vi "Str_Data.vi"(1 "Err str":string, 2 "Msg":T1 {"ID" format="%x"; "MSGTYPE" items=["STATUS"=128, "EXTENDED"=2, "RTR"=1, "DATA MSG"=0]; "aDATA" format="%x"}, 3 "string":string) -> (0 "str out":string)   [LabVIEW 2010]
panel:
  out "str out 2":string
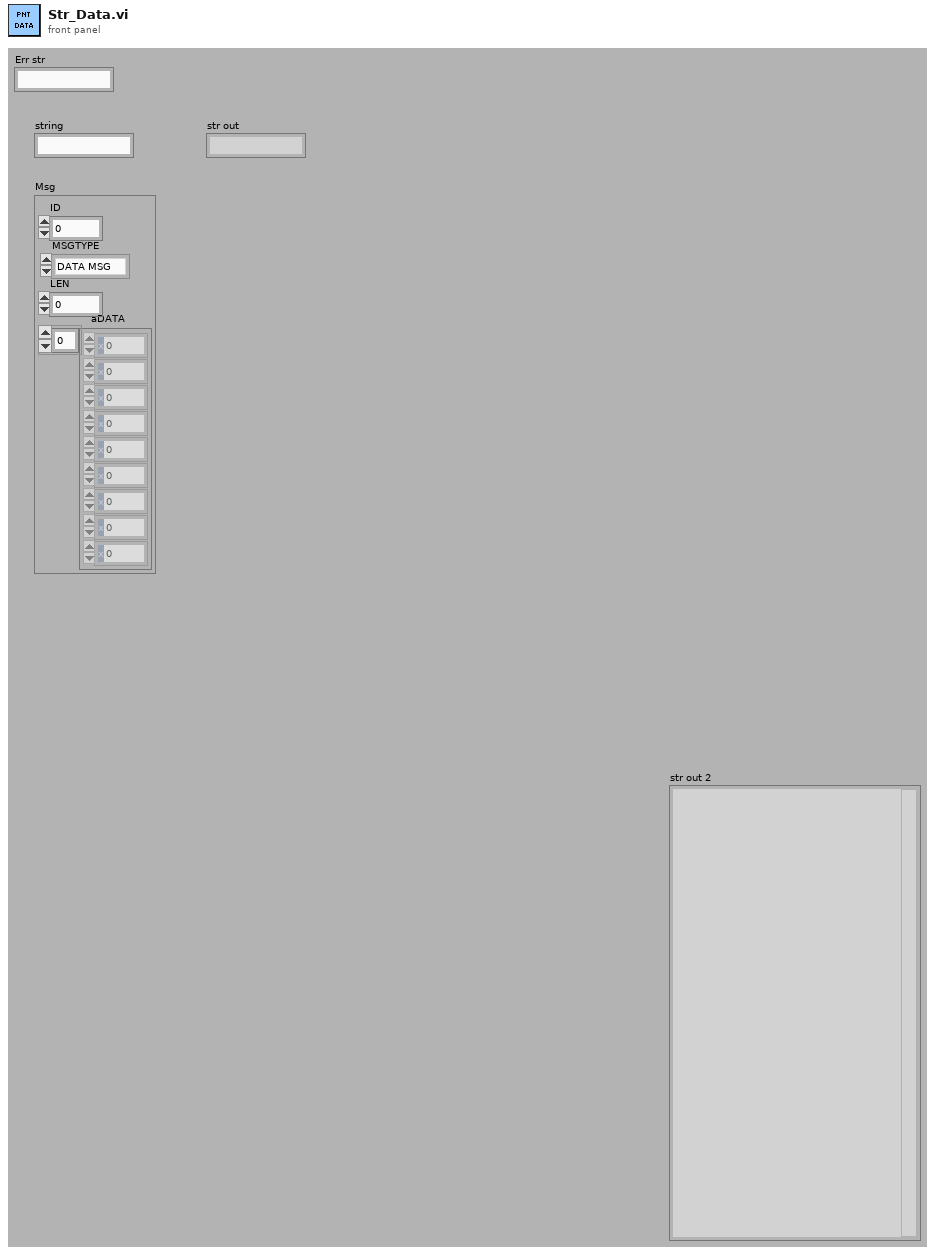
[diagram p1: front panel]
types:
  T1 = cluster{"ID":u32, "MSGTYPE":u8, "LEN":u8, "aDATA":u8[]}
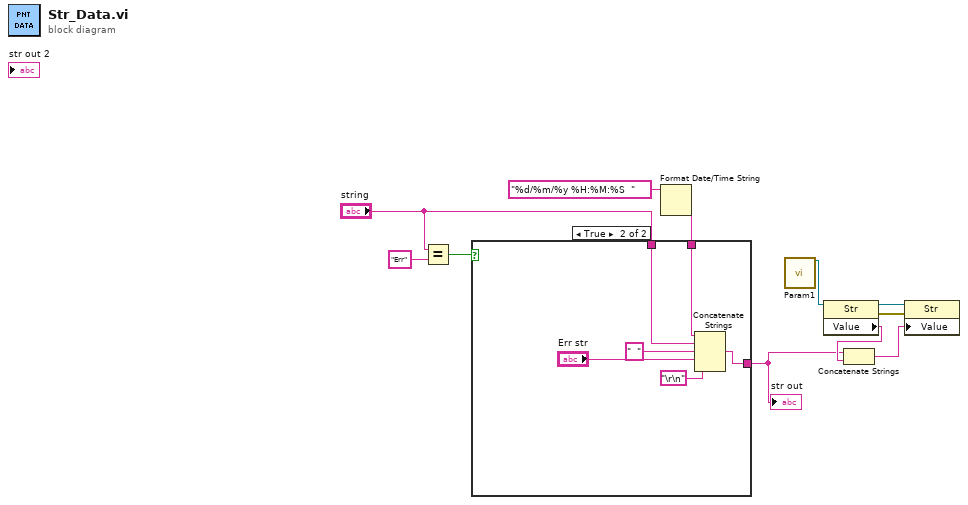
[diagram p0: block diagram]
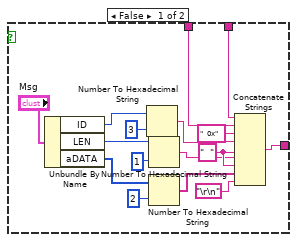
[diagram p2: hidden frame]
diagram:
  n1 = Equal?(x="string", y="Err") -> (x = y?=w1:bool)
  n2 = Format Date/Time String(time format string (%c)="%d/%m/%y %H:%M:%S  ") -> (date/time string=w11:string)  [unwired: 2 in]
  n3 = case shown="True" w1 {
    tunnel: w11 -> [w20 w32]
    tunnel: [w14 w33] -> w4
    tunnel: "string" -> [w13 w31]
    frame False {
      w24 = "  " ("string")
      n4 = Unbundle By Name("Msg") -> ("ID"=w16:u32, "LEN"=w17:u8, "aDATA"=w25:u8[])
      n5 = Number To Hexadecimal String(1:i16 3 ("width (-)"), 2:w16) -> (0:w22:string)
      n6 = Number To Hexadecimal String(1:i16 1 ("width (-)"), 2:w17) -> (0:w23:string)
      n7 = Number To Hexadecimal String(1:i16 2 ("width (-)"), 2:w25) -> (0:w26:string[])
      n8 = Concatenate Strings(w20, w13, "  0x" ("string"), w22, w24, w23, w24, w26, "\r\n") -> (w14:string)
    }
    frame True {
      n9 = Concatenate Strings(w32, w31, "  " ("string"), "Err str", "\r\n") -> (w33:string)
    }
  }
  "str out" <- w4
  n10 = call "Param1.vi"() -> ("str out"=w5:refnum<vi>)  [unwired: 18 in, 1 out]
  n11 = property class="Str"(reference=w5) -> (reference out=w8:refnum<vi>, error out=w7:errorcluster, "Value"=w9:string)  [unwired: 1 in]
  n12 = Concatenate Strings(w4, w9) -> (w6:string)
  n13 = property class="Str"(reference=w8, error in=w7, "Value"=w6) -> ()  [unwired: 2 out]
